vi "Close Local Event Log.vi"(8 "error in (no error)":errorcluster, 10 "Deferred Close Time (0 ms)":u32, 11 "Logger in":refnum<class "Logger.lvclass">) -> (0 "error out":errorcluster, 3 "Logger out":refnum<class "Logger.lvclass">)   [LabVIEW 2020, in "Event Log.lvlib" / "Logger.lvclass"]
uses:
  Logger.lvclass
  Logger.lvclass/Logger.ctl
  <vilib>/gpm_packages/@cs/event-logger/Source/Composed Log/LoggerReference/LoggerReference.lvclass
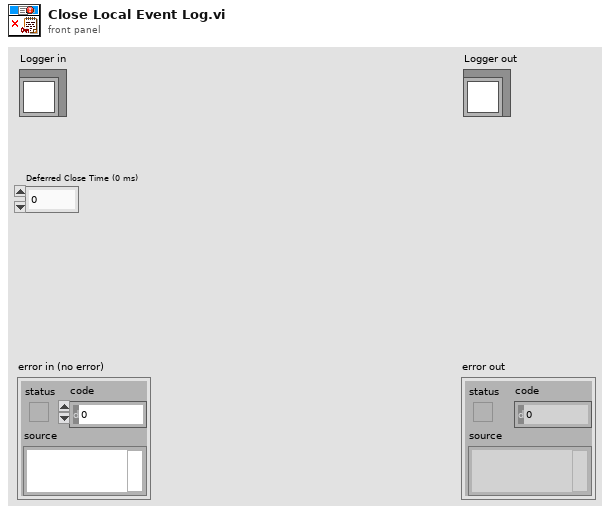
[diagram p1: front panel]
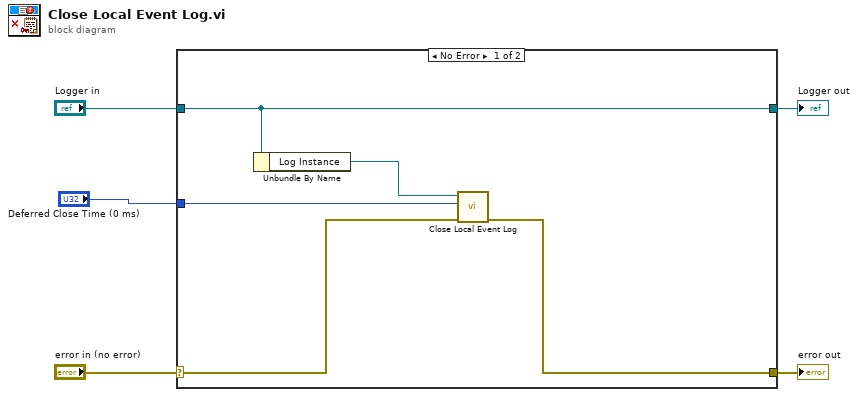
[diagram p0: block diagram]
diagram:
  n1 = case shown="No Error" "error in (no error)" {
    selector: "error in (no error)" -> [w8 w12]
    tunnel: [w7 w12] -> w4
    tunnel: [w10 w11] -> w2
    tunnel: "Logger in" -> [w10 w11]
    tunnel: "Deferred Close Time (0 ms)" -> [w6 _]
    frame No Error {
      n2 = Unbundle By Name(w10) -> ("Log Instance"=w9:refnum<class "LoggerReference.lvclass">)
      n3 = call <vilib>:"Close Local Event Log.vi"("error in (no error)"=w8, "Deferred Close Time (0 ms)"=w6, "Log Instance"=w9) -> ("error out"=w7:errorcluster)  [unwired: 8 in]
    }
    frame Error {
    }
  }
  "error out" <- w4
  "Logger out" <- w2
